vi "broadbandInput.vi"() -> ()   [LabVIEW 2020]
uses:
  <vilib>/Simulation/Scripting/Companion Diagram/SimConfigNode/SimParams.ctl
  <vilib>/Simulation/Scripting/Companion Diagram/SimConfigNode/_simSolvers.ctl
  <vilib>/Simulation/Implementation/Shared/SIMSCR Execution Mode.ctl
  <vilib>/Simulation/Param Hierarchy/Typedefs/SIMPH Param Control Actions.ctl
  <vilib>/Simulation/Implementation/Shared/NILVSim_ParamChanged.vi
  <vilib>/Simulation/Implementation/Shared/NILVSim_FinishedLate.vi
  <vilib>/Simulation/Implementation/Shared/NILVSIM_BeginStep.vi
  <vilib>/Simulation/Utility/Implementation/SIM Time.vi
  <vilib>/Simulation/SignalDisplay/Implementation/NILVSim Time Waveform.llb/SIM Time Waveform (vector).vi
  <vilib>/Simulation/Implementation/Shared/NILVSim_Manager.vi
  <vilib>/Utility/error.llb/Clear Errors.vi
  <vilib>/Simulation/Implementation/Shared/NILVSim_FinalizeModel.vi
  <vilib>/Simulation/Implementation/Shared/SIM Unbundle Sim Info.vi
  <vilib>/Simulation/Implementation/Shared/SIMSH Read Queue.vi
  <vilib>/Simulation/Implementation/Shared/NILVSim_Initialize.vi
  <vilib>/Simulation/Utility/Implementation/NILVSim Get Time and IsAcceptedStep.vi
  <vilib>/Simulation/Implementation/Shared/NILVSim_GetModelError.vi
  <vilib>/Simulation/Implementation/Shared/SIM Bundle Sim Info.vi
  <vilib>/Waveform/WDTOps.llb/WDT Get Waveform Time Array DBL.vi
  <vilib>/Simulation/Scripting/Companion Diagram/SimConfigNode/SimDog.xnode
  Dependencies/sumOfFrequencies.vi
  Dependencies/binary_approx_sumOfFrequencies.vi
  Dependencies/noise_and_binaryNoise.vi
  Dependencies/pseudorandomBinaryNoise (PRBS) and MLS dependencies/PRBS_bit_generator_indexer.vi
  <vilib>/Simulation/Implementation/XNodeFramework/SimXNode/SimX.xnode
  <vilib>/measure/NI_MABase.lvlib
  <vilib>/Simulation/Implementation/Shared/NI_SIM_Implementation.lvlib
panel:
  in  "Bit Size\n(how long is the sequence)":i64=96
  out "MLS value at Index":u8
  in  "MLS array index\n\nNote: start from 0":i32
  out "Which Bit are we at?":dbl
  out "simulation time":dbl
  in  "sampling info":cluster{"Fs":dbl, "#s":dbl}={"Fs"=1000.0, "#s"=1000.0} {"Fs" format="%.2p"}
  out "Waveform Chart 2":u8[](graph)
  in  "stop":bool
  out "X array":timestamp[](array[timestamp])
  out "Noise and Binary Noise":waveform(dbl)[](graph)
  out "Noise":dbl
  out "Binary Noise":dbl
  out "output \nBinary Sum of frequencies":dbl
  out "output":dbl
  out "Waveform Chart":waveform(dbl)[](graph)
  in  "signal type":enum16{"Sine", "Square", "Sawtooth", "Random"}(ring)
  in  "amplitude":dbl=1.0
  in  "frequency":dbl=0.5
  in  "offset":dbl
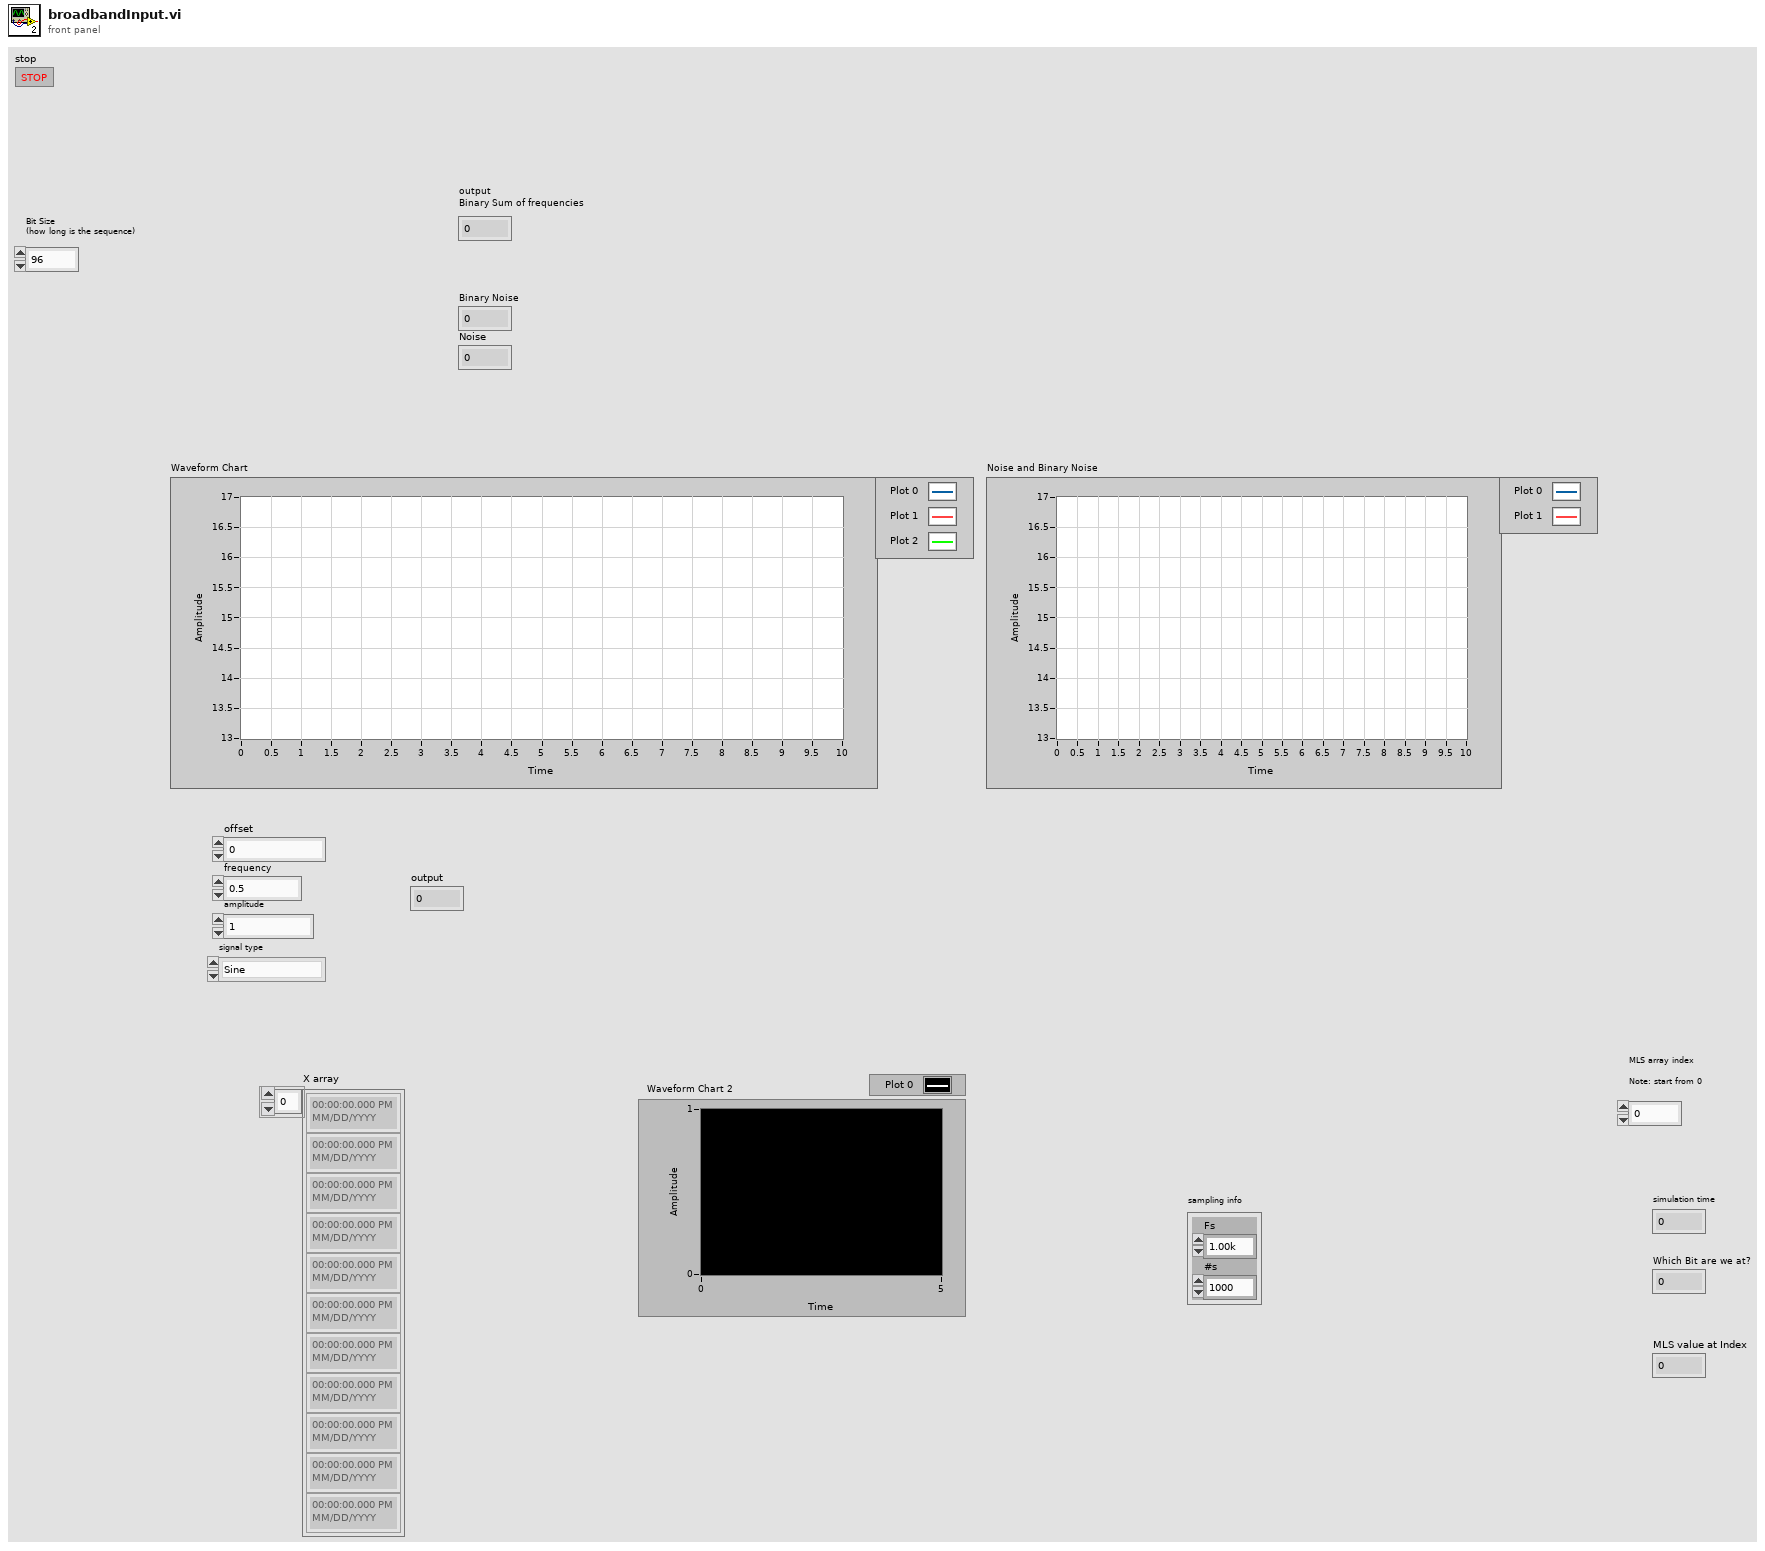
[diagram p1: front panel]
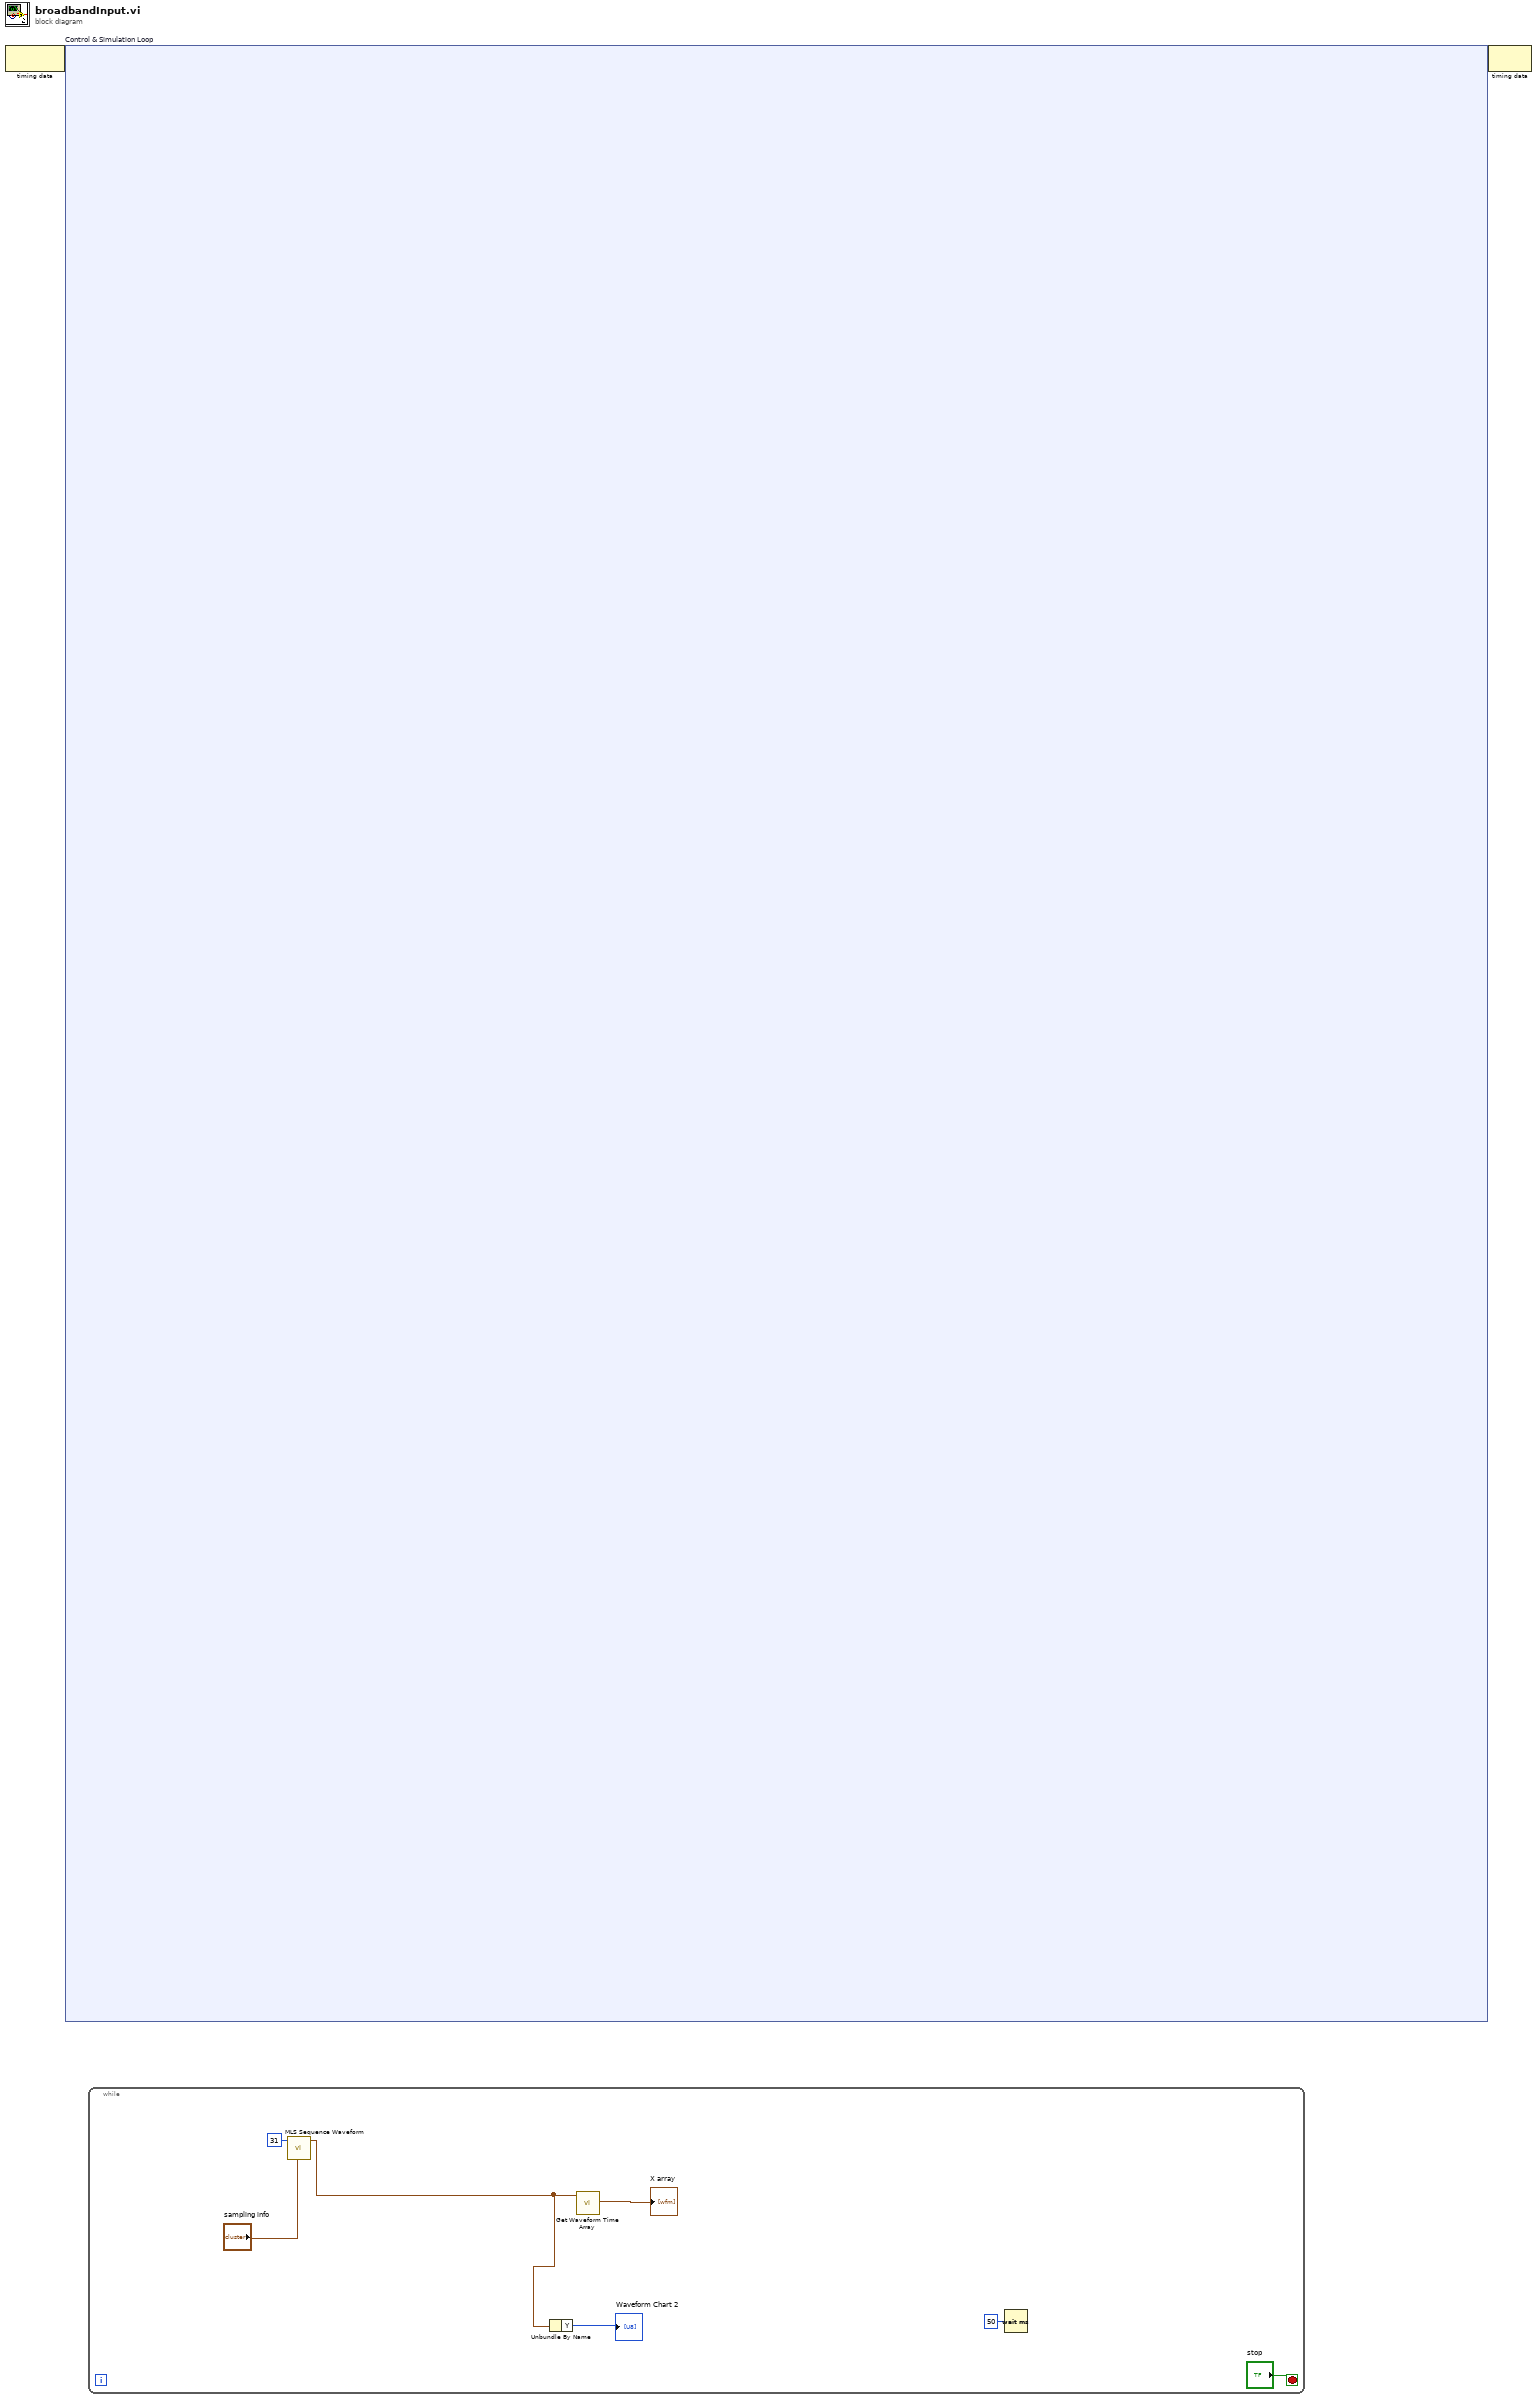
[diagram p0: block diagram]
diagram:
  n1 = node-c288() -> (w2:variant)  [unwired: 1 in]
  n2 = node-c254 "Control & Simulation Loop"(w2) -> (w1:variant)
  n3 = while {
    stop <- "stop" stop-if-true
    n4 = call <vilib>:"MLS Sequence Waveform.vi"("sampling info"="sampling info", "polynomial order"=31) -> ("signal out"=w4:waveform(u8))  [unwired: 8 in, 1 out]
    n5 = Unbundle By Name(w4) -> ("Y"=→"Waveform Chart 2":u8[])
    n6 = call-poly <vilib>:"Get Waveform Time Array.vi"("waveform in"=w4) -> ("X array"=→"X array":timestamp[])  [unwired: 9 in, 1 out]
    n7 = Wait (ms)(milliseconds to wait=u32 50) -> ()  [unwired: 1 out]
  }
  n8 = node-c288(w1) -> ()  [unwired: 1 out]
